vi "MultiDeviceDServer.vi"() -> ()   [LabVIEW 2014, in "examples.lvlib"]
uses:
  examples.lvlib
  vis/tango_vi.llb/_DServerClientRequest.ctl
  vis/tango_vi.llb/_DServerClientRequestType.ctl
  vis/tango_vi.llb/_DServerClientRequestData.ctl
  vis/tango_vi.llb/_GenericDataBuffer.ctl
  vis/tango_vi.llb/_AttributeDataType_t.ctl
  vis/tango_vi.llb/_TangoState_t.ctl
  vis/tango_vi.llb/_DServerSetStateScalarAttributeValue.vi
  vis/tango_vi.llb/_DServerSetStringScalarAttributeValue.vi
  Common/UtilsRandomInstances/_UtilsRandom2DBoolArray.vi
  vis/tango_vi.llb/_DServerSetBooleanImageAttributeValue.vi
  Common/UtilsRandomInstances/_UtilsRandomBoolValue.vi
  vis/tango_vi.llb/_DServerSetBooleanScalarAttributeValue.vi
  Common/UtilsRandomInstances/_UtilsRandomBoolArray.vi
  vis/tango_vi.llb/_DServerSetBooleanSpectrumAttributeValue.vi
  Common/UtilsRandomInstances/_UtilsRandom2DDBLArray.vi
  vis/tango_vi.llb/_DServerSetDoubleImageAttributeValue.vi
  vis/tango_vi.llb/_DServerSetDoubleScalarAttributeValue.vi
  Common/UtilsRandomInstances/_UtilsRandomDBLArray.vi
  vis/tango_vi.llb/_DServerSetDoubleSpectrumAttributeValue.vi
  Common/UtilsRandomInstances/_UtilsRandom2DSGLArray.vi
  vis/tango_vi.llb/_DServerSetFloatImageAttributeValue.vi
  Common/UtilsRandomInstances/_UtilsRandomSGLArray.vi
  vis/tango_vi.llb/_DServerSetFloatSpectrumAttributeValue.vi
  Common/UtilsRandomInstances/_UtilsRandom2DU64Array.vi
  vis/tango_vi.llb/_DServerSetLong64ImageAttributeValue.vi
  Common/UtilsRandomInstances/_UtilsRandomI64Value.vi
  vis/tango_vi.llb/_DServerSetLong64ScalarAttributeValue.vi
  Common/UtilsRandomInstances/_UtilsRandomI64Array.vi
  vis/tango_vi.llb/_DServerSetLong64SpectrumAttributeValue.vi
  Common/UtilsRandomInstances/_UtilsRandom2DI32Array.vi
  vis/tango_vi.llb/_DServerSetLongImageAttributeValue.vi
  Common/UtilsRandomInstances/_UtilsRandomI32Value.vi
  vis/tango_vi.llb/_DServerSetLongScalarAttributeValue.vi
  Common/UtilsRandomInstances/_UtilsRandomU32Array.vi
  vis/tango_vi.llb/_DServerSetLongSpectrumAttributeValue.vi
  Common/UtilsRandomInstances/_UtilsRandom2DI16Array.vi
  vis/tango_vi.llb/_DServerSetShortImageAttributeValue.vi
  Common/UtilsRandomInstances/_UtilsRandomI16Value.vi
  vis/tango_vi.llb/_DServerSetEnumScalarAttributeValue.vi
  Common/UtilsRandomInstances/_UtilsRandomI16Array.vi
  vis/tango_vi.llb/_DServerSetShortSpectrumAttributeValue.vi
  vis/tango_vi.llb/_DServerSetStateImageAttributeValue.vi
  vis/tango_vi.llb/_DServerSetStateSpectrumAttributeValue.vi
  vis/tango_vi.llb/_DServerSetStringImageAttributeValue.vi
  vis/tango_vi.llb/_DServerSetStringSpectrumAttributeValue.vi
  Common/UtilsRandomInstances/_UtilsRandom2DU8Array.vi
  vis/tango_vi.llb/_DServerSetUCharImageAttributeValue.vi
  Common/UtilsRandomInstances/_UtilsRandomU8Value.vi
  vis/tango_vi.llb/_DServerSetUCharScalarAttributeValue.vi
  Common/UtilsRandomInstances/_UtilsRandomU8Array.vi
  vis/tango_vi.llb/_DServerSetUCharSpectrumAttributeValue.vi
  Common/UtilsRandomInstances/_UtilsRandom2DI64Array.vi
  Common/UtilsRandomInstances/_UtilsRandomU64Value.vi
  vis/tango_vi.llb/_DServerSetULong64ScalarAttributeValue.vi
  Common/UtilsRandomInstances/_UtilsRandomU64Array.vi
  vis/tango_vi.llb/_DServerSetULong64SpectrumAttributeValue.vi
  Common/UtilsRandomInstances/_UtilsRandom2DU32Array.vi
  vis/tango_vi.llb/_DServerSetULongImageAttributeValue.vi
  Common/UtilsRandomInstances/_UtilsRandomU32Value.vi
  vis/tango_vi.llb/_DServerSetULongScalarAttributeValue.vi
  Common/UtilsRandomInstances/_UtilsRandomI32Array.vi
  vis/tango_vi.llb/_DServerSetULongSpectrumAttributeValue.vi
  Common/UtilsRandomInstances/_UtilsRandom2DU16Array.vi
  vis/tango_vi.llb/_DServerSetUShortImageAttributeValue.vi
  Common/UtilsRandomInstances/_UtilsRandomU16Value.vi
  vis/tango_vi.llb/_DServerSetUShortScalarAttributeValue.vi
  Common/UtilsRandomInstances/_UtilsRandomU16Array.vi
  vis/tango_vi.llb/_DServerSetUShortSpectrumAttributeValue.vi
  vis/tango_vi.llb/tango.lvlib
panel:
  out "Tango Device State 2.1":T1=enum."UNKNOWN"
  out "Tango Device State 1.2":T1=enum."UNKNOWN"
  in  "devDoubleScalar":dbl(knob)=70.0 scale=0.0..100.0
  out "labview/device/2.1":T2={"Request Id"=0, "Source Id"=0, "Request Type"=enum."UNKNOWN_REQUEST", "Device Class Name"="unspecified/device/name", "Device Name"="unspecified/device/name", "Cmd or Attr Name"="unspecified_cmd_or_attr_name", "Client Request Data"={"write attribute value"={"dimx"=0, "dimy"=0, "data"=[], "data_type"=enum."UNKNOWN_DATA_TYPE"}, "exec. command argin"={"num data"=[], "str data"=[]}}}
  in  "devDoubleScalar":dbl(knob)=50.0 scale=0.0..100.0
  out "Tango Device State 1.1":T1=enum."UNKNOWN"
  out "labview/device/1.2":T2={"Request Id"=0, "Source Id"=0, "Request Type"=enum."UNKNOWN_REQUEST", "Device Class Name"="unspecified/device/name", "Device Name"="unspecified/device/name", "Cmd or Attr Name"="unspecified_cmd_or_attr_name", "Client Request Data"={"write attribute value"={"dimx"=0, "dimy"=0, "data"=[], "data_type"=enum."UNKNOWN_DATA_TYPE"}, "exec. command argin"={"num data"=[], "str data"=[]}}}
  out "labview/device/1.1":T2={"Request Id"=0, "Source Id"=0, "Request Type"=enum."UNKNOWN_REQUEST", "Device Class Name"="unspecified/device/name", "Device Name"="unspecified/device/name", "Cmd or Attr Name"="unspecified_cmd_or_attr_name", "Client Request Data"={"write attribute value"={"dimx"=0, "dimy"=0, "data"=[], "data_type"=enum."UNKNOWN_DATA_TYPE"}, "exec. command argin"={"num data"=[], "str data"=[]}}}
  in  "Tango Client Request":T2={"Request Id"=0, "Source Id"=0, "Request Type"=enum."UNKNOWN_REQUEST", "Device Class Name"="unspecified_class_name", "Device Name"="unspecified/device/name", "Cmd or Attr Name"="unspecified_cmd_or_attr_name", "Client Request Data"={"write attribute value"={"dimx"=0, "dimy"=0, "data"=[], "data_type"=enum."UNKNOWN_DATA_TYPE"}, "exec. command argin"={"num data"=[], "str data"=[]}}}
  out "Device List":string[](array[string])
  in  "Instance Name":string="1"
  in  "Executable Name":string="LabviewMultiDeviceDServer"
  in  "devDoubleScalar":dbl(knob)=30.0 scale=0.0..100.0
  in  "?":bool
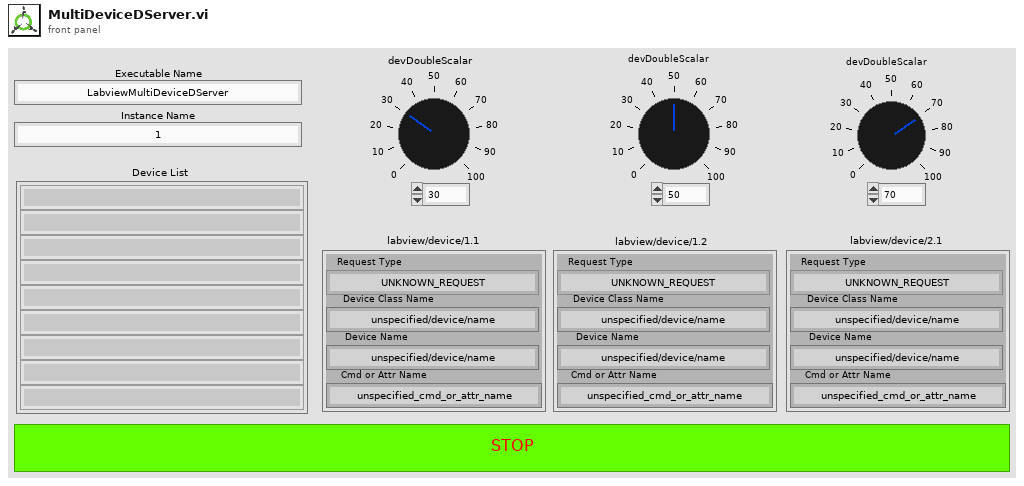
[diagram p1: front panel]
types:
  T1 = typedef "tango.lvlib/_TangoState_t.ctl" = enum32{"ON", "OFF", "CLOSE", "OPEN", "INSERT", "EXTRACT", "MOVING", "STANDBY", "FAULT", "INIT", "RUNNING", "ALARM", "DISABLE", "UNKNOWN"}
  T2 = typedef "tango.lvlib/_DServerClientRequest.ctl" = cluster{"Request Id":u32, "Source Id":u32, "Request Type":T3, "Device Class Name":string, "Device Name":string, "Cmd or Attr Name":string, "Client Request Data":T4}
  T3 = typedef "tango.lvlib/_DServerClientRequestType.ctl" = enum16{"EXEC_CMD", "READ_ATTR", "WRITE_ATTR", "UNKNOWN_REQUEST"}
  T4 = typedef "tango.lvlib/_DServerClientRequestData.ctl" = cluster{"write attribute value":T5, "exec. command argin":cluster{"num data":u8[], "str data":string[]}}
  T5 = typedef "tango.lvlib/_GenericDataBuffer.ctl" = cluster{"dimx":u32, "dimy":u32, "data":u8[], "data_type":T6}
  T6 = typedef "tango.lvlib/_AttributeDataType_t.ctl" = enum16{"STATE_SCA", "STATE_SPE", "STATE_IMG", "STRING_SCA", "STRING_SPE", "STRING_IMG", "BOOL_SCA", "BOOL_SPE", "BOOL_IMG", "UCHAR_SCA", "UCHAR_SPE", "UCHAR_IMG", "SHORT_SCA", "SHORT_SPE", "SHORT_IMG", "USHORT_SCA", "USHORT_SPE", "USHORT_IMG", "LONG_SCA", "LONG_SPE", "LONG_IMG", "ULONG_SCA", "ULONG_SPE", "ULONG_IMG", "LONG64_SCA", "LONG64_SPE", "LONG64_IMG", "ULONG64_SCA", "ULONG64_SPE", "ULONG64_IMG", "FLOAT_SCA", "FLOAT_SPE", "FLOAT_IMG", "DOUBLE_SCA", "DOUBLE_SPE", "DOUBLE_IMG", "ENUM_SCA", "UNKNOWN_DATA_TYPE"}
  T7 = typedef "tango.lvlib/_DServerEvent.ctl" = cluster{"event registration refnum":refnum<event-registration>, "user event out":refnum<user-event>}
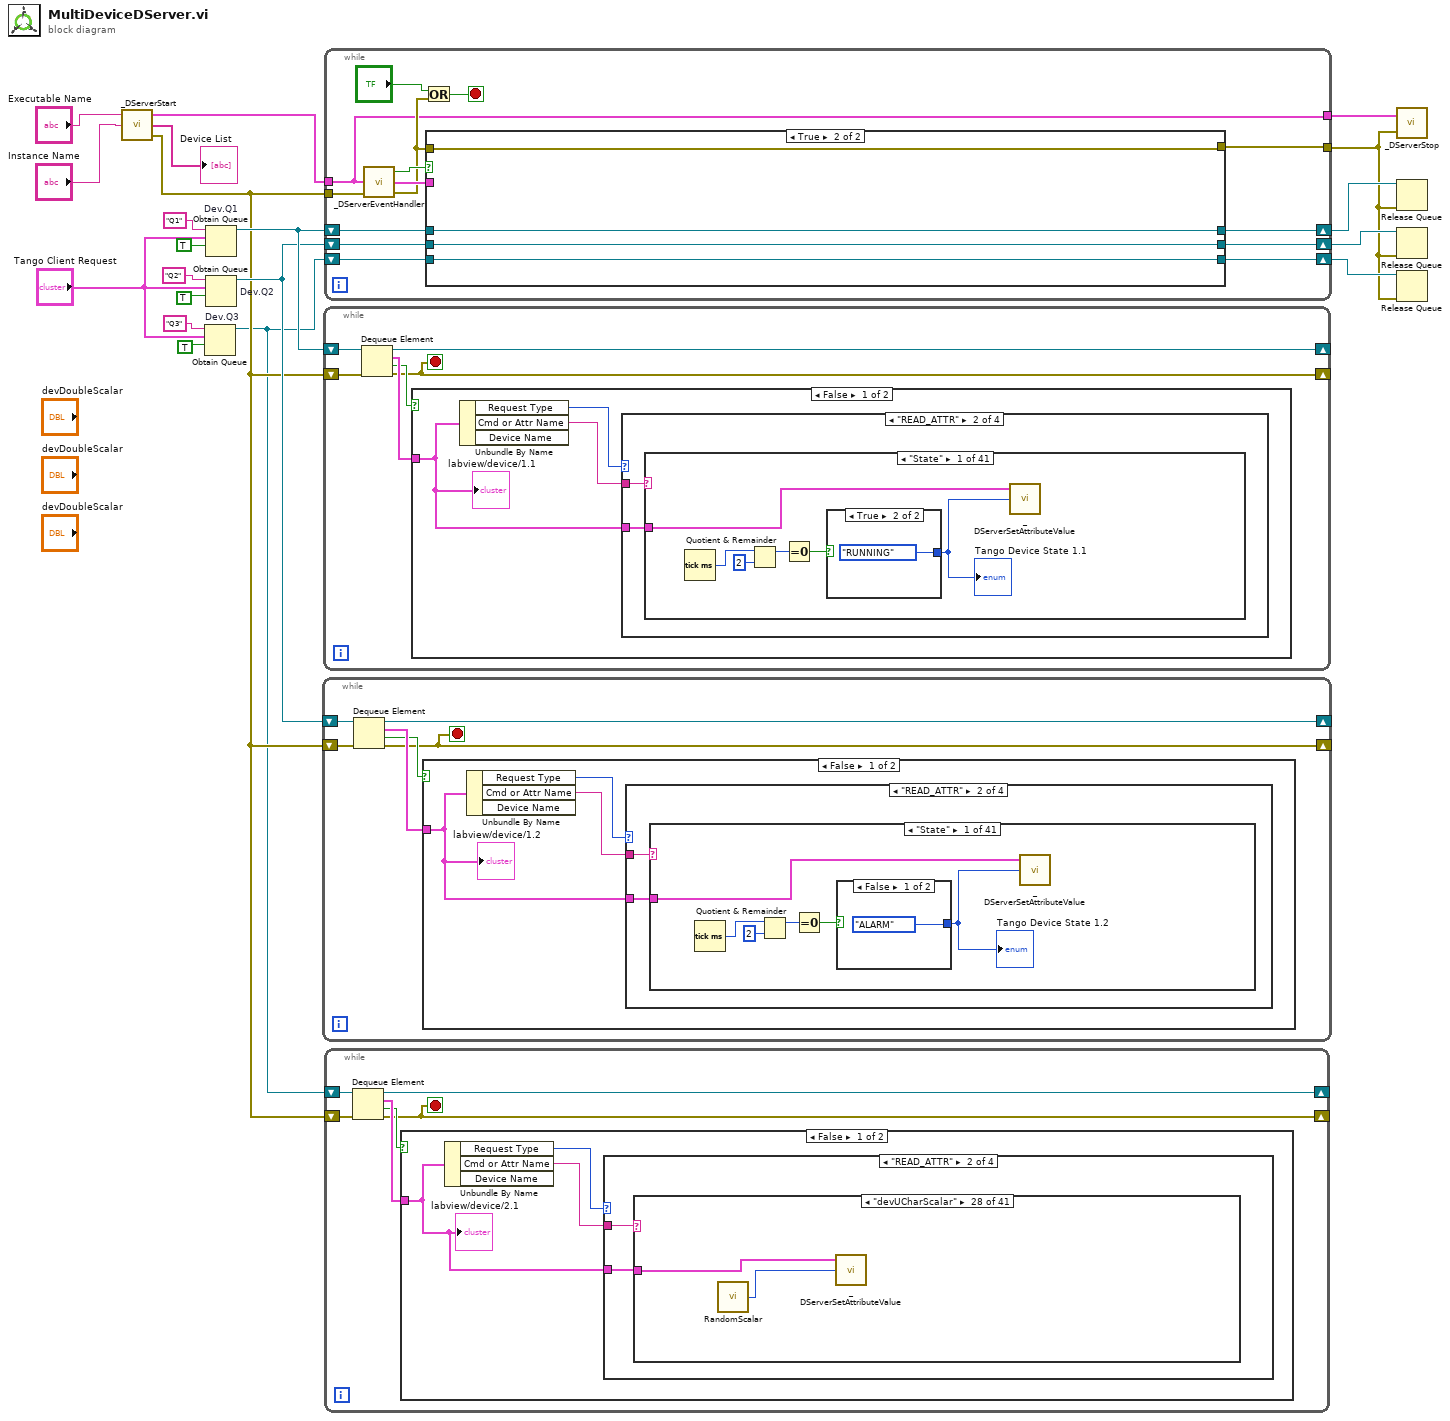
[diagram p0: block diagram]
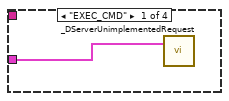
[diagram p2: hidden frame]
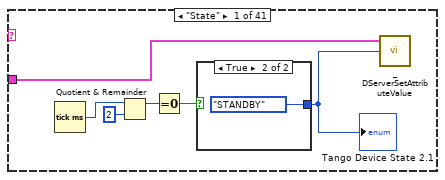
[diagram p3: hidden frame]
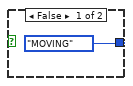
[diagram p4: hidden frame]
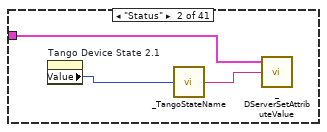
[diagram p5: hidden frame]
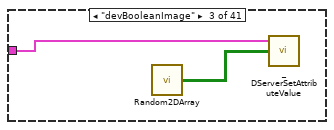
[diagram p6: hidden frame]
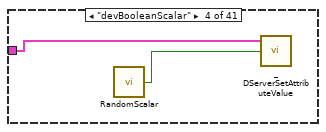
[diagram p7: hidden frame]
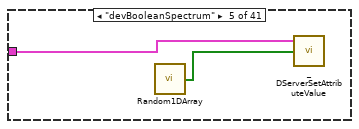
[diagram p8: hidden frame]
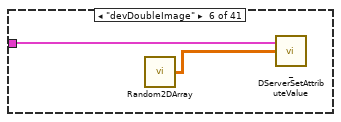
[diagram p9: hidden frame]
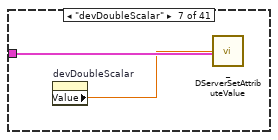
[diagram p10: hidden frame]
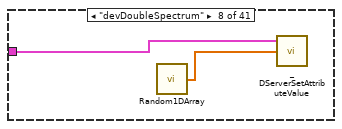
[diagram p11: hidden frame]
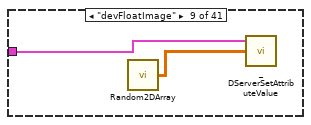
[diagram p12: hidden frame]
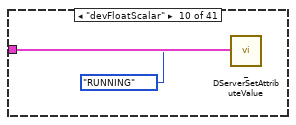
[diagram p13: hidden frame]
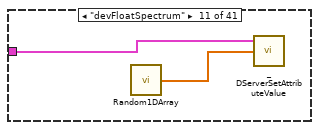
[diagram p14: hidden frame]
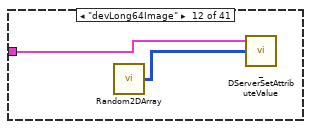
[diagram p15: hidden frame]
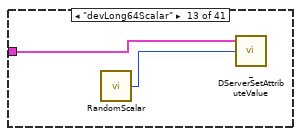
[diagram p16: hidden frame]
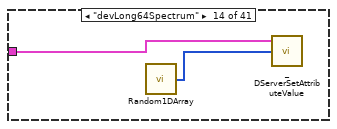
[diagram p17: hidden frame]
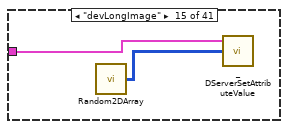
[diagram p18: hidden frame]
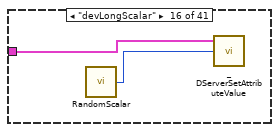
[diagram p19: hidden frame]
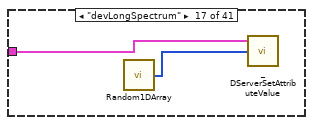
[diagram p20: hidden frame]
diagram:
  n1 = call "_DServerStart.vi"("instance name"="Instance Name", "executable name"="Executable Name") -> ("error out"=w2:errorcluster, "device_list"=→"Device List":string[], "dserver evt."=w5:T7)  [unwired: 1 in]
  n2 = Obtain Queue "Dev.Q3"(name (unnamed)="Q3", element data type="Tango Client Request", create if not found? (T)=TRUE) -> (queue out=w1:refnum<queue>)  [unwired: 2 in, 2 out]
  n3 = Obtain Queue "Dev.Q1"(name (unnamed)="Q1", element data type="Tango Client Request", create if not found? (T)=TRUE) -> (queue out=w18:refnum<queue>)  [unwired: 2 in, 2 out]
  n4 = Obtain Queue "Dev.Q2"(name (unnamed)="Q2", element data type="Tango Client Request", create if not found? (T)=TRUE) -> (queue out=w14:refnum<queue>)  [unwired: 2 in, 2 out]
  n5 = while {
    shift-right: [w21] -> _
    shift-left: w2 -> [w22]
    shift-right: [w23] -> _
    shift-left: w14 -> [w26]
    stop <- w21 stop-if-true
    n6 = Dequeue Element(queue=w26, error in (no error)=w22) -> (queue out=w23:refnum<queue>, element=w25:T2, timed out?=w24:bool, error out=w21:errorcluster)  [unwired: 1 in]
    n7 = case shown="False" w24 {
      tunnel: w25 -> [w27 _]
      frame False {
        n8 = Unbundle By Name(w27) -> ("Request Type"=w28:T3, "Cmd or Attr Name"=w29:string)  [unwired: 1 out]
        n9 = case shown="\"READ_ATTR\"" w28 {
          tunnel: w29 -> [_ w32 _ _]
          tunnel: w27 -> [w30 w31 w140 w141]
          frame "EXEC_CMD" {
            n10 = call "_DServerUnimplementedRequest.vi"("client request"=w30) -> ()  [unwired: 2 in, 1 out]
          }
          frame "READ_ATTR" {
            n11 = case shown="\"State\"" w32 {
              tunnel: w31 -> [w34 w42 w45 w47 w49 w51 w53 w55 w57 w58 w61 w63 w65 w67 w69 w71 w73 w75 w77 w79 w82 w85 w95 w102 w105 w110 w112 w114 w116 w118 w120 w122 w124 w126 w128 w130 w132 w134 w135 _ w139]
              frame "State" {
                n12 = Tick Count (ms)() -> (millisecond timer value=w35:u32)
                n13 = Quotient & Remainder(x=w35, y=u32 2) -> (x-y*floor(x/y)=w37:u32)  [unwired: 1 out]
                n14 = Equal To 0?(x=w37) -> (x = 0?=w36:bool)
                n15 = case shown="False" w36 {
                  tunnel: [_TangoState_t."ALARM" ("Tango Device State") _TangoState_t."FAULT" ("Tango Device State")] -> w33
                  frame False {
                  }
                  frame True {
                  }
                }
                "Tango Device State 1.2" <- w33
                n16 = call-poly "_DServerSetAttributeValue.vi"("value"=w33, "client request"=w34) -> ()  [unwired: 3 in, 1 out]
              }
              frame "Status" {
                n17 = property on="Tango Device State 1.2" class="Enum (strict)"() -> ("Value"=w41:T1)  [unwired: 2 in, 2 out]
                n18 = call "_TangoStateName.vi"("State"=w41) -> ("State Name"=w43:string)
                n19 = call-poly "_DServerSetAttributeValue.vi"("value"=w43, "client request"=w42) -> ()  [unwired: 3 in, 1 out]
              }
              frame "devBooleanImage" {
                n20 = call-poly "Random2DArray.vi"() -> ("random array"=w44:bool[][])  [unwired: 2 in]
                n21 = call-poly "_DServerSetAttributeValue.vi"("value"=w44, "client request"=w45) -> ()  [unwired: 3 in, 1 out]
              }
              frame "devBooleanScalar" {
                n22 = call-poly "RandomScalar.vi"() -> ("random value"=w46:bool)  [unwired: 1 in]
                n23 = call-poly "_DServerSetAttributeValue.vi"(4:w46, "client request"=w47) -> ()  [unwired: 3 in, 1 out]
              }
              frame "devBooleanSpectrum" {
                n24 = call-poly "Random1DArray.vi"() -> ("array"=w48:bool[])  [unwired: 2 in]
                n25 = call-poly "_DServerSetAttributeValue.vi"("value"=w48, "client request"=w49) -> ()  [unwired: 3 in, 1 out]
              }
              frame "devDoubleImage" {
                n26 = call-poly "Random2DArray.vi"() -> ("random array"=w50:dbl[][])  [unwired: 2 in]
                n27 = call-poly "_DServerSetAttributeValue.vi"("value"=w50, "client request"=w51) -> ()  [unwired: 3 in, 1 out]
              }
              frame "devDoubleScalar" {
                n28 = property on="devDoubleScalar" class="Knob (strict)"() -> ("Value"=w52:dbl)  [unwired: 2 in, 2 out]
                n29 = call-poly "_DServerSetAttributeValue.vi"("value"=w52, "client request"=w53) -> ()  [unwired: 3 in, 1 out]
              }
              frame "devDoubleSpectrum" {
                n30 = call-poly "Random1DArray.vi"() -> ("array"=w54:dbl[])  [unwired: 2 in]
                n31 = call-poly "_DServerSetAttributeValue.vi"("value"=w54, "client request"=w55) -> ()  [unwired: 3 in, 1 out]
              }
              frame "devFloatImage" {
                n32 = call-poly "Random2DArray.vi"() -> ("random array"=w56:sgl[][])  [unwired: 2 in]
                n33 = call-poly "_DServerSetAttributeValue.vi"("value"=w56, "client request"=w57) -> ()  [unwired: 3 in, 1 out]
              }
              frame "devFloatScalar" {
                n34 = call-poly "_DServerSetAttributeValue.vi"("value"=_TangoState_t."RUNNING" ("Tango Device State"), "client request"=w58) -> ()  [unwired: 3 in, 1 out]
              }
              frame "devFloatSpectrum" {
                n35 = call-poly "Random1DArray.vi"() -> ("array"=w60:sgl[])  [unwired: 2 in]
                n36 = call-poly "_DServerSetAttributeValue.vi"("value"=w60, "client request"=w61) -> ()  [unwired: 3 in, 1 out]
              }
              frame "devLong64Image" {
                n37 = call-poly "Random2DArray.vi"() -> ("random array"=w62:i64[][])  [unwired: 2 in]
                n38 = call-poly "_DServerSetAttributeValue.vi"("value"=w62, "client request"=w63) -> ()  [unwired: 3 in, 1 out]
              }
              frame "devLong64Scalar" {
                n39 = call-poly "RandomScalar.vi"() -> ("random value"=w64:i64)  [unwired: 1 in]
                n40 = call-poly "_DServerSetAttributeValue.vi"("value"=w64, "client request"=w65) -> ()  [unwired: 3 in, 1 out]
              }
              frame "devLong64Spectrum" {
                n41 = call-poly "Random1DArray.vi"() -> ("array"=w66:i64[])  [unwired: 2 in]
                n42 = call-poly "_DServerSetAttributeValue.vi"("value"=w66, "client request"=w67) -> ()  [unwired: 3 in, 1 out]
              }
              frame "devLongImage" {
                n43 = call-poly "Random2DArray.vi"() -> ("random array"=w68:i32[][])  [unwired: 2 in]
                n44 = call-poly "_DServerSetAttributeValue.vi"("value"=w68, "client request"=w69) -> ()  [unwired: 3 in, 1 out]
              }
              frame "devLongScalar" {
                n45 = call-poly "RandomScalar.vi"() -> ("random value"=w70:i32)  [unwired: 1 in]
                n46 = call-poly "_DServerSetAttributeValue.vi"("value"=w70, "client request"=w71) -> ()  [unwired: 3 in, 1 out]
              }
              frame "devLongSpectrum" {
                n47 = call-poly "Random1DArray.vi"() -> ("array"=w72:i32[])  [unwired: 2 in]
                n48 = call-poly "_DServerSetAttributeValue.vi"("value"=w72, "client request"=w73) -> ()  [unwired: 3 in, 1 out]
              }
              frame "devShortImage" {
                n49 = call-poly "Random2DArray.vi"() -> ("random array"=w74:i16[][])  [unwired: 2 in]
                n50 = call-poly "_DServerSetAttributeValue.vi"("value"=w74, "client request"=w75) -> ()  [unwired: 3 in, 1 out]
              }
              frame "devShortScalar" {
                n51 = call-poly "RandomScalar.vi"() -> ("random value"=w76:i16)  [unwired: 1 in]
                n52 = call-poly "_DServerSetAttributeValue.vi"("value"=w76, "client request"=w77) -> ()  [unwired: 3 in, 1 out]
              }
              frame "devShortSpectrum" {
                n53 = call-poly "Random1DArray.vi"() -> ("array"=w78:i16[])  [unwired: 2 in]
                n54 = call-poly "_DServerSetAttributeValue.vi"("value"=w78, "client request"=w79) -> ()  [unwired: 3 in, 1 out]
              }
              frame "devStateImage" {
                n55 = property on="Tango Device State 1.2" class="Enum (strict)"() -> ("Value"=w81:T1)  [unwired: 2 in, 2 out]
                n56 = Initialize Array(w81, 32 ("dimension size"), 32 ("dimension size")) -> (w80:T1[][])
                n57 = call-poly "_DServerSetAttributeValue.vi"("value"=w80, "client request"=w82) -> ()  [unwired: 3 in, 1 out]
              }
              frame "devStateScalar" {
                n58 = Tick Count (ms)() -> (millisecond timer value=w87:u32)
                n59 = Quotient & Remainder(x=w87, y=u32 2) -> (x-y*floor(x/y)=w89:u32)  [unwired: 1 out]
                n60 = Equal To 0?(x=w89) -> (x = 0?=w88:bool)
                n61 = case shown="False" w88 {
                  tunnel: [_TangoState_t."STANDBY" ("Tango Device State") _TangoState_t."RUNNING" ("Tango Device State")] -> w86
                  frame False {
                  }
                  frame True {
                  }
                }
                n62 = call-poly "_DServerSetAttributeValue.vi"("value"=w86, "client request"=w85) -> ()  [unwired: 3 in, 1 out]
              }
              frame "devStateSpectrum" {
                n63 = property on="Tango Device State 1.2" class="Enum (strict)"() -> ("Value"=w94:T1)  [unwired: 2 in, 2 out]
                n64 = Initialize Array(w94, 32 ("dimension size")) -> (w93:T1[])
                n65 = call-poly "_DServerSetAttributeValue.vi"("value"=w93, "client request"=w95) -> ()  [unwired: 3 in, 1 out]
              }
              frame "devStringImage" {
                n66 = call "RandomValue.vi"() -> ("random value"=w100:dbl)  [unwired: 1 in]
                n67 = Number To Hexadecimal String(2:w100) -> (0:w99:string)  [unwired: 1 in]
                n68 = Initialize Array(w99, 32 ("dimension size"), 32 ("dimension size")) -> (w98:string[][])
                n69 = call-poly "_DServerSetAttributeValue.vi"("value"=w98, "client request"=w102) -> ()  [unwired: 3 in, 1 out]
              }
              frame "devStringScalar" {
                n70 = call "RandomValue.vi"() -> ("random value"=w104:dbl)  [unwired: 1 in]
                n71 = Number To Hexadecimal String(2:w104) -> (0:w103:string)  [unwired: 1 in]
                n72 = call-poly "_DServerSetAttributeValue.vi"("value"=w103, "client request"=w105) -> ()  [unwired: 3 in, 1 out]
              }
              frame "devStringSpectrum" {
                n73 = call "RandomValue.vi"() -> ("random value"=w108:dbl)  [unwired: 1 in]
                n74 = Number To Hexadecimal String(2:w108) -> (0:w107:string)  [unwired: 1 in]
                n75 = Initialize Array(w107, 32 ("dimension size")) -> (w106:string[])
                n76 = call-poly "_DServerSetAttributeValue.vi"("value"=w106, "client request"=w110) -> ()  [unwired: 3 in, 1 out]
              }
              frame "devUCharImage" {
                n77 = call-poly "Random2DArray.vi"() -> ("random array"=w111:u8[][])  [unwired: 2 in]
                n78 = call-poly "_DServerSetAttributeValue.vi"("value"=w111, "client request"=w112) -> ()  [unwired: 3 in, 1 out]
              }
              frame "devUCharScalar" {
                n79 = call-poly "RandomScalar.vi"() -> ("random value"=w113:u8)  [unwired: 1 in]
                n80 = call-poly "_DServerSetAttributeValue.vi"("value"=w113, "client request"=w114) -> ()  [unwired: 3 in, 1 out]
              }
              frame "devUCharSpectrum" {
                n81 = call-poly "Random1DArray.vi"() -> ("array"=w115:u8[])  [unwired: 2 in]
                n82 = call-poly "_DServerSetAttributeValue.vi"("value"=w115, "client request"=w116) -> ()  [unwired: 3 in, 1 out]
              }
              frame "devULong64Image" {
                n83 = call-poly "Random2DArray.vi"() -> ("random array"=w117:i64[][])  [unwired: 2 in]
                n84 = call-poly "_DServerSetAttributeValue.vi"("value"=w117, "client request"=w118) -> ()  [unwired: 3 in, 1 out]
              }
              frame "devULong64Scalar" {
                n85 = call-poly "RandomScalar.vi"() -> ("random value"=w119:u64)  [unwired: 1 in]
                n86 = call-poly "_DServerSetAttributeValue.vi"("value"=w119, "client request"=w120) -> ()  [unwired: 3 in, 1 out]
              }
              frame "devULong64Spectrum" {
                n87 = call-poly "Random1DArray.vi"() -> ("array"=w121:u64[])  [unwired: 2 in]
                n88 = call-poly "_DServerSetAttributeValue.vi"("value"=w121, "client request"=w122) -> ()  [unwired: 3 in, 1 out]
              }
              frame "devULongImage" {
                n89 = call-poly "Random2DArray.vi"() -> ("random array"=w123:u32[][])  [unwired: 2 in]
                n90 = call-poly "_DServerSetAttributeValue.vi"("value"=w123, "client request"=w124) -> ()  [unwired: 3 in, 1 out]
              }
              frame "devULongScalar" {
                n91 = call-poly "RandomScalar.vi"() -> ("random value"=w125:u32)  [unwired: 1 in]
                n92 = call-poly "_DServerSetAttributeValue.vi"("value"=w125, "client request"=w126) -> ()  [unwired: 3 in, 1 out]
              }
              frame "devULongSpectrum" {
                n93 = call-poly "Random1DArray.vi"() -> ("array"=w127:u32[])  [unwired: 2 in]
                n94 = call-poly "_DServerSetAttributeValue.vi"("value"=w127, "client request"=w128) -> ()  [unwired: 3 in, 1 out]
              }
              frame "devUShortImage" {
                n95 = call-poly "Random2DArray.vi"() -> ("random array"=w129:u16[][])  [unwired: 2 in]
                n96 = call-poly "_DServerSetAttributeValue.vi"("value"=w129, "client request"=w130) -> ()  [unwired: 3 in, 1 out]
              }
              frame "devUShortScalar" {
                n97 = call-poly "RandomScalar.vi"() -> ("random value"=w131:u16)  [unwired: 1 in]
                n98 = call-poly "_DServerSetAttributeValue.vi"("value"=w131, "client request"=w132) -> ()  [unwired: 3 in, 1 out]
              }
              frame "devUShortSpectrum" {
                n99 = call-poly "Random1DArray.vi"() -> ("array"=w133:u16[])  [unwired: 2 in]
                n100 = call-poly "_DServerSetAttributeValue.vi"("value"=w133, "client request"=w134) -> ()  [unwired: 3 in, 1 out]
              }
              frame "slowReplyAttribute" {
                n101 = stacked-sequence {
                  tunnel: w135 -> [_ w138]
                  frame #0 {
                    # "simulate a slow reply \ngenerating a client \nrequest timeout"
                    n102 = Wait (ms)(milliseconds to wait=u32 3500) -> ()  [unwired: 1 out]
                  }
                  frame #1 {
                    # "simulate a slow reply \ngenerating a client \nrequest timeout"
                    n103 = call-poly "Random1DArray.vi"() -> ("array"=w137:u8[])  [unwired: 2 in]
                    n104 = call-poly "_DServerSetAttributeValue.vi"("value"=w137, "client request"=w138) -> ()  [unwired: 3 in, 1 out]
                  }
                }
              }
              frame "noReplyAttribute" {
                # "we voluntarily don't reply to this request in order to\nobserve the behavior of the tango binding to such a \nsituation - we expect the waiter (i.e. the thread handling \nthe client request to timeout and leave the place) - the \ntango device will block (i.e. will not be able to handle \nanother request) until the timeout expires - we consequently understand easily why we should reply to any single request - the _DServerUnimplementedRequest.vi can be temporary used to deal with \"not yet implemented\" features - see the \"unhandledAttribute\" case for an example"
              }
              frame "unHandledAttribute", Default {
                n105 = call "_DServerUnimplementedRequest.vi"("client request"=w139) -> ()  [unwired: 2 in, 1 out]
              }
            }
          }
          frame "WRITE_ATTR" {
            n106 = call "_DServerUnimplementedRequest.vi"("client request"=w140) -> ()  [unwired: 2 in, 1 out]
          }
          frame "UNKNOWN_REQUEST", Default {
            n107 = call "_DServerUnimplementedRequest.vi"("client request"=w141) -> ()  [unwired: 2 in, 1 out]
          }
        }
        "labview/device/1.2" <- w27
      }
      frame True {
      }
    }
  }
  n108 = while {
    shift-right: [w142] -> _
    shift-left: w2 -> [w143]
    shift-right: [w144] -> _
    shift-left: w18 -> [w147]
    stop <- w142 stop-if-true
    n109 = Dequeue Element(queue=w147, error in (no error)=w143) -> (queue out=w144:refnum<queue>, element=w146:T2, timed out?=w145:bool, error out=w142:errorcluster)  [unwired: 1 in]
    n110 = case shown="False" w145 {
      tunnel: w146 -> [w148 _]
      frame False {
        n111 = Unbundle By Name(w148) -> ("Request Type"=w149:T3, "Cmd or Attr Name"=w150:string)  [unwired: 1 out]
        n112 = case shown="\"READ_ATTR\"" w149 {
          tunnel: w150 -> [_ w153 _ _]
          tunnel: w148 -> [w151 w152 w261 w262]
          frame "EXEC_CMD" {
            n113 = call "_DServerUnimplementedRequest.vi"("client request"=w151) -> ()  [unwired: 2 in, 1 out]
          }
          frame "READ_ATTR" {
            n114 = case shown="\"State\"" w153 {
              tunnel: w152 -> [w155 w163 w166 w168 w170 w172 w174 w176 w178 w180 w182 w184 w186 w188 w190 w192 w194 w196 w198 w200 w203 w206 w217 w223 w226 w231 w233 w235 w237 w239 w241 w243 w245 w247 w249 w251 w253 w255 w256 _ w260]
              frame "State" {
                n115 = Tick Count (ms)() -> (millisecond timer value=w156:u32)
                n116 = Quotient & Remainder(x=w156, y=u32 2) -> (x-y*floor(x/y)=w158:u32)  [unwired: 1 out]
                n117 = Equal To 0?(x=w158) -> (x = 0?=w157:bool)
                n118 = case shown="True" w157 {
                  tunnel: [_TangoState_t."STANDBY" ("Tango Device State") _TangoState_t."RUNNING" ("Tango Device State")] -> w154
                  frame False {
                  }
                  frame True {
                  }
                }
                "Tango Device State 1.1" <- w154
                n119 = call-poly "_DServerSetAttributeValue.vi"("value"=w154, "client request"=w155) -> ()  [unwired: 3 in, 1 out]
              }
              frame "Status" {
                n120 = property on="Tango Device State 1.1" class="Enum (strict)"() -> ("Value"=w162:T1)  [unwired: 2 in, 2 out]
                n121 = call "_TangoStateName.vi"("State"=w162) -> ("State Name"=w164:string)
                n122 = call-poly "_DServerSetAttributeValue.vi"("value"=w164, "client request"=w163) -> ()  [unwired: 3 in, 1 out]
              }
              frame "devBooleanImage" {
                n123 = call-poly "Random2DArray.vi"() -> ("random array"=w165:bool[][])  [unwired: 2 in]
                n124 = call-poly "_DServerSetAttributeValue.vi"("value"=w165, "client request"=w166) -> ()  [unwired: 3 in, 1 out]
              }
              frame "devBooleanScalar" {
                n125 = call-poly "RandomScalar.vi"() -> ("random value"=w167:bool)  [unwired: 1 in]
                n126 = call-poly "_DServerSetAttributeValue.vi"(4:w167, "client request"=w168) -> ()  [unwired: 3 in, 1 out]
              }
              frame "devBooleanSpectrum" {
                n127 = call-poly "Random1DArray.vi"() -> ("array"=w169:bool[])  [unwired: 2 in]
                n128 = call-poly "_DServerSetAttributeValue.vi"("value"=w169, "client request"=w170) -> ()  [unwired: 3 in, 1 out]
              }
              frame "devDoubleImage" {
                n129 = call-poly "Random2DArray.vi"() -> ("random array"=w171:dbl[][])  [unwired: 2 in]
                n130 = call-poly "_DServerSetAttributeValue.vi"("value"=w171, "client request"=w172) -> ()  [unwired: 3 in, 1 out]
              }
              frame "devDoubleScalar" {
                n131 = property on="devDoubleScalar" class="Knob (strict)"() -> ("Value"=w173:dbl)  [unwired: 2 in, 2 out]
                n132 = call-poly "_DServerSetAttributeValue.vi"("value"=w173, "client request"=w174) -> ()  [unwired: 3 in, 1 out]
              }
              frame "devDoubleSpectrum" {
                n133 = call-poly "Random1DArray.vi"() -> ("array"=w175:dbl[])  [unwired: 2 in]
                n134 = call-poly "_DServerSetAttributeValue.vi"("value"=w175, "client request"=w176) -> ()  [unwired: 3 in, 1 out]
              }
              frame "devFloatImage" {
                n135 = call-poly "Random2DArray.vi"() -> ("random array"=w177:sgl[][])  [unwired: 2 in]
                n136 = call-poly "_DServerSetAttributeValue.vi"("value"=w177, "client request"=w178) -> ()  [unwired: 3 in, 1 out]
              }
              frame "devFloatScalar" {
                n137 = call-poly "_DServerSetAttributeValue.vi"("value"=_TangoState_t."RUNNING" ("Tango Device State"), "client request"=w180) -> ()  [unwired: 3 in, 1 out]
              }
              frame "devFloatSpectrum" {
                n138 = call-poly "Random1DArray.vi"() -> ("array"=w181:sgl[])  [unwired: 2 in]
                n139 = call-poly "_DServerSetAttributeValue.vi"("value"=w181, "client request"=w182) -> ()  [unwired: 3 in, 1 out]
              }
              frame "devLong64Image" {
                n140 = call-poly "Random2DArray.vi"() -> ("random array"=w183:i64[][])  [unwired: 2 in]
                n141 = call-poly "_DServerSetAttributeValue.vi"("value"=w183, "client request"=w184) -> ()  [unwired: 3 in, 1 out]
              }
              frame "devLong64Scalar" {
                n142 = call-poly "RandomScalar.vi"() -> ("random value"=w185:i64)  [unwired: 1 in]
                n143 = call-poly "_DServerSetAttributeValue.vi"("value"=w185, "client request"=w186) -> ()  [unwired: 3 in, 1 out]
              }
              frame "devLong64Spectrum" {
                n144 = call-poly "Random1DArray.vi"() -> ("array"=w187:i64[])  [unwired: 2 in]
                n145 = call-poly "_DServerSetAttributeValue.vi"("value"=w187, "client request"=w188) -> ()  [unwired: 3 in, 1 out]
              }
              frame "devLongImage" {
                n146 = call-poly "Random2DArray.vi"() -> ("random array"=w189:i32[][])  [unwired: 2 in]
                n147 = call-poly "_DServerSetAttributeValue.vi"("value"=w189, "client request"=w190) -> ()  [unwired: 3 in, 1 out]
              }
              frame "devLongScalar" {
                n148 = call-poly "RandomScalar.vi"() -> ("random value"=w191:i32)  [unwired: 1 in]
                n149 = call-poly "_DServerSetAttributeValue.vi"("value"=w191, "client request"=w192) -> ()  [unwired: 3 in, 1 out]
              }
              frame "devLongSpectrum" {
                n150 = call-poly "Random1DArray.vi"() -> ("array"=w193:i32[])  [unwired: 2 in]
                n151 = call-poly "_DServerSetAttributeValue.vi"("value"=w193, "client request"=w194) -> ()  [unwired: 3 in, 1 out]
              }
              frame "devShortImage" {
                n152 = call-poly "Random2DArray.vi"() -> ("random array"=w195:i16[][])  [unwired: 2 in]
                n153 = call-poly "_DServerSetAttributeValue.vi"("value"=w195, "client request"=w196) -> ()  [unwired: 3 in, 1 out]
              }
              frame "devShortScalar" {
                n154 = call-poly "RandomScalar.vi"() -> ("random value"=w197:i16)  [unwired: 1 in]
                n155 = call-poly "_DServerSetAttributeValue.vi"("value"=w197, "client request"=w198) -> ()  [unwired: 3 in, 1 out]
              }
              frame "devShortSpectrum" {
                n156 = call-poly "Random1DArray.vi"() -> ("array"=w199:i16[])  [unwired: 2 in]
                n157 = call-poly "_DServerSetAttributeValue.vi"("value"=w199, "client request"=w200) -> ()  [unwired: 3 in, 1 out]
              }
              frame "devStateImage" {
                n158 = property on="Tango Device State 1.1" class="Enum (strict)"() -> ("Value"=w201:T1)  [unwired: 2 in, 2 out]
                n159 = Initialize Array(w201, 32 ("dimension size"), 32 ("dimension size")) -> (w202:T1[][])
                n160 = call-poly "_DServerSetAttributeValue.vi"("value"=w202, "client request"=w203) -> ()  [unwired: 3 in, 1 out]
              }
              frame "devStateScalar" {
                n161 = Tick Count (ms)() -> (millisecond timer value=w208:u32)
                n162 = Quotient & Remainder(x=w208, y=u32 2) -> (x-y*floor(x/y)=w210:u32)  [unwired: 1 out]
                n163 = Equal To 0?(x=w210) -> (x = 0?=w209:bool)
                n164 = case shown="False" w209 {
                  tunnel: [_TangoState_t."STANDBY" ("Tango Device State") _TangoState_t."RUNNING" ("Tango Device State")] -> w207
                  frame False {
                  }
                  frame True {
                  }
                }
                n165 = call-poly "_DServerSetAttributeValue.vi"("value"=w207, "client request"=w206) -> ()  [unwired: 3 in, 1 out]
              }
              frame "devStateSpectrum" {
                n166 = property on="Tango Device State 1.1" class="Enum (strict)"() -> ("Value"=w216:T1)  [unwired: 2 in, 2 out]
                n167 = Initialize Array(w216, 32 ("dimension size")) -> (w214:T1[])
                n168 = call-poly "_DServerSetAttributeValue.vi"("value"=w214, "client request"=w217) -> ()  [unwired: 3 in, 1 out]
              }
              frame "devStringImage" {
                n169 = call "RandomValue.vi"() -> ("random value"=w221:dbl)  [unwired: 1 in]
                n170 = Number To Hexadecimal String(2:w221) -> (0:w220:string)  [unwired: 1 in]
                n171 = Initialize Array(w220, 32 ("dimension size"), 32 ("dimension size")) -> (w219:string[][])
                n172 = call-poly "_DServerSetAttributeValue.vi"("value"=w219, "client request"=w223) -> ()  [unwired: 3 in, 1 out]
              }
              frame "devStringScalar" {
                n173 = call "RandomValue.vi"() -> ("random value"=w225:dbl)  [unwired: 1 in]
                n174 = Number To Hexadecimal String(2:w225) -> (0:w224:string)  [unwired: 1 in]
                n175 = call-poly "_DServerSetAttributeValue.vi"("value"=w224, "client request"=w226) -> ()  [unwired: 3 in, 1 out]
              }
              frame "devStringSpectrum" {
                n176 = call "RandomValue.vi"() -> ("random value"=w229:dbl)  [unwired: 1 in]
                n177 = Number To Hexadecimal String(2:w229) -> (0:w228:string)  [unwired: 1 in]
                n178 = Initialize Array(w228, 32 ("dimension size")) -> (w227:string[])
                n179 = call-poly "_DServerSetAttributeValue.vi"("value"=w227, "client request"=w231) -> ()  [unwired: 3 in, 1 out]
              }
              frame "devUCharImage" {
                n180 = call-poly "Random2DArray.vi"() -> ("random array"=w232:u8[][])  [unwired: 2 in]
                n181 = call-poly "_DServerSetAttributeValue.vi"("value"=w232, "client request"=w233) -> ()  [unwired: 3 in, 1 out]
              }
              frame "devUCharScalar" {
                n182 = call-poly "RandomScalar.vi"() -> ("random value"=w234:u8)  [unwired: 1 in]
                n183 = call-poly "_DServerSetAttributeValue.vi"("value"=w234, "client request"=w235) -> ()  [unwired: 3 in, 1 out]
              }
              frame "devUCharSpectrum" {
                n184 = call-poly "Random1DArray.vi"() -> ("array"=w236:u8[])  [unwired: 2 in]
                n185 = call-poly "_DServerSetAttributeValue.vi"("value"=w236, "client request"=w237) -> ()  [unwired: 3 in, 1 out]
              }
              frame "devULong64Image" {
                n186 = call-poly "Random2DArray.vi"() -> ("random array"=w238:i64[][])  [unwired: 2 in]
                n187 = call-poly "_DServerSetAttributeValue.vi"("value"=w238, "client request"=w239) -> ()  [unwired: 3 in, 1 out]
              }
              frame "devULong64Scalar" {
                n188 = call-poly "RandomScalar.vi"() -> ("random value"=w240:u64)  [unwired: 1 in]
                n189 = call-poly "_DServerSetAttributeValue.vi"("value"=w240, "client request"=w241) -> ()  [unwired: 3 in, 1 out]
              }
              frame "devULong64Spectrum" {
                n190 = call-poly "Random1DArray.vi"() -> ("array"=w242:u64[])  [unwired: 2 in]
                n191 = call-poly "_DServerSetAttributeValue.vi"("value"=w242, "client request"=w243) -> ()  [unwired: 3 in, 1 out]
              }
              frame "devULongImage" {
                n192 = call-poly "Random2DArray.vi"() -> ("random array"=w244:u32[][])  [unwired: 2 in]
                n193 = call-poly "_DServerSetAttributeValue.vi"("value"=w244, "client request"=w245) -> ()  [unwired: 3 in, 1 out]
              }
              frame "devULongScalar" {
                n194 = call-poly "RandomScalar.vi"() -> ("random value"=w246:u32)  [unwired: 1 in]
                n195 = call-poly "_DServerSetAttributeValue.vi"("value"=w246, "client request"=w247) -> ()  [unwired: 3 in, 1 out]
              }
              frame "devULongSpectrum" {
                n196 = call-poly "Random1DArray.vi"() -> ("array"=w248:u32[])  [unwired: 2 in]
                n197 = call-poly "_DServerSetAttributeValue.vi"("value"=w248, "client request"=w249) -> ()  [unwired: 3 in, 1 out]
              }
              frame "devUShortImage" {
                n198 = call-poly "Random2DArray.vi"() -> ("random array"=w250:u16[][])  [unwired: 2 in]
                n199 = call-poly "_DServerSetAttributeValue.vi"("value"=w250, "client request"=w251) -> ()  [unwired: 3 in, 1 out]
              }
              frame "devUShortScalar" {
                n200 = call-poly "RandomScalar.vi"() -> ("random value"=w252:u16)  [unwired: 1 in]
                n201 = call-poly "_DServerSetAttributeValue.vi"("value"=w252, "client request"=w253) -> ()  [unwired: 3 in, 1 out]
              }
              frame "devUShortSpectrum" {
                n202 = call-poly "Random1DArray.vi"() -> ("array"=w254:u16[])  [unwired: 2 in]
                n203 = call-poly "_DServerSetAttributeValue.vi"("value"=w254, "client request"=w255) -> ()  [unwired: 3 in, 1 out]
              }
              frame "slowReplyAttribute" {
                n204 = stacked-sequence {
                  tunnel: w256 -> [_ w259]
                  frame #0 {
                    # "simulate a slow reply \ngenerating a client \nrequest timeout"
                    n205 = Wait (ms)(milliseconds to wait=u32 3500) -> ()  [unwired: 1 out]
                  }
                  frame #1 {
                    # "simulate a slow reply \ngenerating a client \nrequest timeout"
                    n206 = call-poly "Random1DArray.vi"() -> ("array"=w258:u8[])  [unwired: 2 in]
                    n207 = call-poly "_DServerSetAttributeValue.vi"("value"=w258, "client request"=w259) -> ()  [unwired: 3 in, 1 out]
                  }
                }
              }
              frame "noReplyAttribute" {
                # "we voluntarily don't reply to this request in order to\nobserve the behavior of the tango binding to such a \nsituation - we expect the waiter (i.e. the thread handling \nthe client request to timeout and leave the place) - the \ntango device will block (i.e. will not be able to handle \nanother request) until the timeout expires - we consequently understand easily why we should reply to any single request - the _DServerUnimplementedRequest.vi can be temporary used to deal with \"not yet implemented\" features - see the \"unhandledAttribute\" case for an example"
              }
              frame "unHandledAttribute", Default {
                n208 = call "_DServerUnimplementedRequest.vi"("client request"=w260) -> ()  [unwired: 2 in, 1 out]
              }
            }
          }
          frame "WRITE_ATTR" {
            n209 = call "_DServerUnimplementedRequest.vi"("client request"=w261) -> ()  [unwired: 2 in, 1 out]
          }
          frame "UNKNOWN_REQUEST", Default {
            n210 = call "_DServerUnimplementedRequest.vi"("client request"=w262) -> ()  [unwired: 2 in, 1 out]
          }
        }
        "labview/device/1.1" <- w148
      }
      frame True {
      }
    }
  }
  n211 = while {
    tunnel: w2 -> [w266]
    tunnel: [w265] -> w3
    shift-right: [w275] -> w17
    shift-left: w18 -> [w276]
    shift-right: [w273] -> w15
    shift-left: w14 -> [w274]
    shift-right: [w270] -> w8
    shift-left: w1 -> [w271]
    tunnel: w5 -> [w263]
    tunnel: [w263] -> w4
    stop <- w272 stop-if-true
    n212 = call "_DServerEventHandler.vi"("error in"=w266, "dserver evt."=w263) -> ("error out"=w267:errorcluster, "client request"=w268:T2, "timeout"=w269:bool)  [unwired: 1 in]
    n213 = Or(x="?", y=w267) -> (x .or. y?=w272:bool)
    n214 = case shown="True" w269 {
      tunnel: w268 -> [w280 _]
      tunnel: w276 -> [w286 w315]
      tunnel: [w281 w315] -> w275
      tunnel: w274 -> [w284 w314]
      tunnel: [w285 w314] -> w273
      tunnel: w271 -> [w283 w313]
      tunnel: [w282 w313] -> w270
      tunnel: w267 -> [w278 w312]
      tunnel: [w277 w312] -> w265
      frame False {
        n215 = Unbundle By Name(w280) -> ("Device Name"=w279:string)
        n216 = case shown="\"labview/device/1.1\"" w279 {
          tunnel: w286 -> [w290 w297 w304 w310]
          tunnel: w284 -> [w289 w296 w302 w311]
          tunnel: [w289 w296 w301 w311] -> w285
          tunnel: [w288 w295 w303 w308] -> w282
          tunnel: w283 -> [w288 w295 w303 w309]
          tunnel: [w290 w294 w304 w310] -> w281
          tunnel: w280 -> [_ w293 w300 w307]
          tunnel: w278 -> [w287 w292 w299 w306]
          tunnel: [w287 w291 w298 w305] -> w277
          frame Default {
          }
          frame "labview/device/1.1" {
            n217 = Enqueue Element(queue=w297, element=w293, error in (no error)=w292) -> (queue out=w294:refnum<queue>, error out=w291:errorcluster)  [unwired: 1 in, 1 out]
          }
          frame "labview/device/1.2" {
            n218 = Enqueue Element(queue=w302, element=w300, error in (no error)=w299) -> (queue out=w301:refnum<queue>, error out=w298:errorcluster)  [unwired: 1 in, 1 out]
          }
          frame "labview/device/2.1" {
            n219 = Enqueue Element(queue=w309, element=w307, error in (no error)=w306) -> (queue out=w308:refnum<queue>, error out=w305:errorcluster)  [unwired: 1 in, 1 out]
          }
        }
      }
      frame True {
      }
    }
  }
  n220 = while {
    shift-right: [w316] -> _
    shift-left: w2 -> [w317]
    shift-right: [w318] -> _
    shift-left: w1 -> [w321]
    stop <- w316 stop-if-true
    n221 = Dequeue Element(queue=w321, error in (no error)=w317) -> (queue out=w318:refnum<queue>, element=w320:T2, timed out?=w319:bool, error out=w316:errorcluster)  [unwired: 1 in]
    n222 = case shown="False" w319 {
      tunnel: w320 -> [w322 _]
      frame False {
        n223 = Unbundle By Name(w322) -> ("Request Type"=w323:T3, "Cmd or Attr Name"=w324:string)  [unwired: 1 out]
        n224 = case shown="\"READ_ATTR\"" w323 {
          tunnel: w324 -> [_ w327 _ _]
          tunnel: w322 -> [w325 w326 w434 w435]
          frame "EXEC_CMD" {
            n225 = call "_DServerUnimplementedRequest.vi"("client request"=w325) -> ()  [unwired: 2 in, 1 out]
          }
          frame "READ_ATTR" {
            n226 = case shown="\"devUCharScalar\"" w327 {
              tunnel: w326 -> [w329 w337 w340 w341 w344 w346 w348 w350 w352 w354 w356 w358 w360 w362 w364 w366 w368 w370 w372 w374 w377 w380 w390 w397 w400 w405 w407 w409 w411 w413 w415 w417 w419 w421 w423 w425 w427 w428 w429 _ w433]
              frame "State" {
                n227 = Tick Count (ms)() -> (millisecond timer value=w330:u32)
                n228 = Quotient & Remainder(x=w330, y=u32 2) -> (x-y*floor(x/y)=w332:u32)  [unwired: 1 out]
                n229 = Equal To 0?(x=w332) -> (x = 0?=w331:bool)
                n230 = case shown="True" w331 {
                  tunnel: [_TangoState_t."MOVING" ("Tango Device State") _TangoState_t."STANDBY" ("Tango Device State")] -> w328
                  frame False {
                  }
                  frame True {
                  }
                }
                "Tango Device State 2.1" <- w328
                n231 = call-poly "_DServerSetAttributeValue.vi"("value"=w328, "client request"=w329) -> ()  [unwired: 3 in, 1 out]
              }
              frame "Status" {
                n232 = property on="Tango Device State 2.1" class="Enum (strict)"() -> ("Value"=w336:T1)  [unwired: 2 in, 2 out]
                n233 = call "_TangoStateName.vi"("State"=w336) -> ("State Name"=w338:string)
                n234 = call-poly "_DServerSetAttributeValue.vi"("value"=w338, "client request"=w337) -> ()  [unwired: 3 in, 1 out]
              }
              frame "devBooleanImage" {
                n235 = call-poly "Random2DArray.vi"() -> ("random array"=w339:bool[][])  [unwired: 2 in]
                n236 = call-poly "_DServerSetAttributeValue.vi"("value"=w339, "client request"=w340) -> ()  [unwired: 3 in, 1 out]
              }
              frame "devBooleanScalar" {
                n237 = call-poly "RandomScalar.vi"() -> ("random value"=w342:bool)  [unwired: 1 in]
                n238 = call-poly "_DServerSetAttributeValue.vi"(4:w342, "client request"=w341) -> ()  [unwired: 3 in, 1 out]
              }
              frame "devBooleanSpectrum" {
                n239 = call-poly "Random1DArray.vi"() -> ("array"=w343:bool[])  [unwired: 2 in]
                n240 = call-poly "_DServerSetAttributeValue.vi"("value"=w343, "client request"=w344) -> ()  [unwired: 3 in, 1 out]
              }
              frame "devDoubleImage" {
                n241 = call-poly "Random2DArray.vi"() -> ("random array"=w345:dbl[][])  [unwired: 2 in]
                n242 = call-poly "_DServerSetAttributeValue.vi"("value"=w345, "client request"=w346) -> ()  [unwired: 3 in, 1 out]
              }
              frame "devDoubleScalar" {
                n243 = property on="devDoubleScalar" class="Knob (strict)"() -> ("Value"=w347:dbl)  [unwired: 2 in, 2 out]
                n244 = call-poly "_DServerSetAttributeValue.vi"("value"=w347, "client request"=w348) -> ()  [unwired: 3 in, 1 out]
              }
              frame "devDoubleSpectrum" {
                n245 = call-poly "Random1DArray.vi"() -> ("array"=w349:dbl[])  [unwired: 2 in]
                n246 = call-poly "_DServerSetAttributeValue.vi"("value"=w349, "client request"=w350) -> ()  [unwired: 3 in, 1 out]
              }
              frame "devFloatImage" {
                n247 = call-poly "Random2DArray.vi"() -> ("random array"=w351:sgl[][])  [unwired: 2 in]
                n248 = call-poly "_DServerSetAttributeValue.vi"("value"=w351, "client request"=w352) -> ()  [unwired: 3 in, 1 out]
              }
              frame "devFloatScalar" {
                n249 = call-poly "_DServerSetAttributeValue.vi"("value"=_TangoState_t."RUNNING" ("Tango Device State"), "client request"=w354) -> ()  [unwired: 3 in, 1 out]
              }
              frame "devFloatSpectrum" {
                n250 = call-poly "Random1DArray.vi"() -> ("array"=w355:sgl[])  [unwired: 2 in]
                n251 = call-poly "_DServerSetAttributeValue.vi"("value"=w355, "client request"=w356) -> ()  [unwired: 3 in, 1 out]
              }
              frame "devLong64Image" {
                n252 = call-poly "Random2DArray.vi"() -> ("random array"=w357:i64[][])  [unwired: 2 in]
                n253 = call-poly "_DServerSetAttributeValue.vi"("value"=w357, "client request"=w358) -> ()  [unwired: 3 in, 1 out]
              }
              frame "devLong64Scalar" {
                n254 = call-poly "RandomScalar.vi"() -> ("random value"=w359:i64)  [unwired: 1 in]
                n255 = call-poly "_DServerSetAttributeValue.vi"("value"=w359, "client request"=w360) -> ()  [unwired: 3 in, 1 out]
              }
              frame "devLong64Spectrum" {
                n256 = call-poly "Random1DArray.vi"() -> ("array"=w361:i64[])  [unwired: 2 in]
                n257 = call-poly "_DServerSetAttributeValue.vi"("value"=w361, "client request"=w362) -> ()  [unwired: 3 in, 1 out]
              }
              frame "devLongImage" {
                n258 = call-poly "Random2DArray.vi"() -> ("random array"=w363:i32[][])  [unwired: 2 in]
                n259 = call-poly "_DServerSetAttributeValue.vi"("value"=w363, "client request"=w364) -> ()  [unwired: 3 in, 1 out]
              }
              frame "devLongScalar" {
                n260 = call-poly "RandomScalar.vi"() -> ("random value"=w365:i32)  [unwired: 1 in]
                n261 = call-poly "_DServerSetAttributeValue.vi"("value"=w365, "client request"=w366) -> ()  [unwired: 3 in, 1 out]
              }
              frame "devLongSpectrum" {
                n262 = call-poly "Random1DArray.vi"() -> ("array"=w367:i32[])  [unwired: 2 in]
                n263 = call-poly "_DServerSetAttributeValue.vi"("value"=w367, "client request"=w368) -> ()  [unwired: 3 in, 1 out]
              }
              frame "devShortImage" {
                n264 = call-poly "Random2DArray.vi"() -> ("random array"=w369:i16[][])  [unwired: 2 in]
                n265 = call-poly "_DServerSetAttributeValue.vi"("value"=w369, "client request"=w370) -> ()  [unwired: 3 in, 1 out]
              }
              frame "devShortScalar" {
                n266 = call-poly "RandomScalar.vi"() -> ("random value"=w371:i16)  [unwired: 1 in]
                n267 = call-poly "_DServerSetAttributeValue.vi"("value"=w371, "client request"=w372) -> ()  [unwired: 3 in, 1 out]
              }
              frame "devShortSpectrum" {
                n268 = call-poly "Random1DArray.vi"() -> ("array"=w373:i16[])  [unwired: 2 in]
                n269 = call-poly "_DServerSetAttributeValue.vi"("value"=w373, "client request"=w374) -> ()  [unwired: 3 in, 1 out]
              }
              frame "devStateImage" {
                n270 = property on="Tango Device State 2.1" class="Enum (strict)"() -> ("Value"=w376:T1)  [unwired: 2 in, 2 out]
                n271 = Initialize Array(w376, 32 ("dimension size"), 32 ("dimension size")) -> (w375:T1[][])
                n272 = call-poly "_DServerSetAttributeValue.vi"("value"=w375, "client request"=w377) -> ()  [unwired: 3 in, 1 out]
              }
              frame "devStateScalar" {
                n273 = Tick Count (ms)() -> (millisecond timer value=w382:u32)
                n274 = Quotient & Remainder(x=w382, y=u32 2) -> (x-y*floor(x/y)=w384:u32)  [unwired: 1 out]
                n275 = Equal To 0?(x=w384) -> (x = 0?=w383:bool)
                n276 = case shown="False" w383 {
                  tunnel: [_TangoState_t."STANDBY" ("Tango Device State") _TangoState_t."RUNNING" ("Tango Device State")] -> w381
                  frame False {
                  }
                  frame True {
                  }
                }
                n277 = call-poly "_DServerSetAttributeValue.vi"("value"=w381, "client request"=w380) -> ()  [unwired: 3 in, 1 out]
              }
              frame "devStateSpectrum" {
                n278 = property on="Tango Device State 2.1" class="Enum (strict)"() -> ("Value"=w389:T1)  [unwired: 2 in, 2 out]
                n279 = Initialize Array(w389, 32 ("dimension size")) -> (w388:T1[])
                n280 = call-poly "_DServerSetAttributeValue.vi"("value"=w388, "client request"=w390) -> ()  [unwired: 3 in, 1 out]
              }
              frame "devStringImage" {
                n281 = call "RandomValue.vi"() -> ("random value"=w395:dbl)  [unwired: 1 in]
                n282 = Number To Hexadecimal String(2:w395) -> (0:w394:string)  [unwired: 1 in]
                n283 = Initialize Array(w394, 32 ("dimension size"), 32 ("dimension size")) -> (w393:string[][])
                n284 = call-poly "_DServerSetAttributeValue.vi"("value"=w393, "client request"=w397) -> ()  [unwired: 3 in, 1 out]
              }
              frame "devStringScalar" {
                n285 = call "RandomValue.vi"() -> ("random value"=w399:dbl)  [unwired: 1 in]
                n286 = Number To Hexadecimal String(2:w399) -> (0:w398:string)  [unwired: 1 in]
                n287 = call-poly "_DServerSetAttributeValue.vi"("value"=w398, "client request"=w400) -> ()  [unwired: 3 in, 1 out]
              }
              frame "devStringSpectrum" {
                n288 = call "RandomValue.vi"() -> ("random value"=w403:dbl)  [unwired: 1 in]
                n289 = Number To Hexadecimal String(2:w403) -> (0:w402:string)  [unwired: 1 in]
                n290 = Initialize Array(w402, 32 ("dimension size")) -> (w401:string[])
                n291 = call-poly "_DServerSetAttributeValue.vi"("value"=w401, "client request"=w405) -> ()  [unwired: 3 in, 1 out]
              }
              frame "devUCharImage" {
                n292 = call-poly "Random2DArray.vi"() -> ("random array"=w406:u8[][])  [unwired: 2 in]
                n293 = call-poly "_DServerSetAttributeValue.vi"("value"=w406, "client request"=w407) -> ()  [unwired: 3 in, 1 out]
              }
              frame "devUCharScalar" {
                n294 = call-poly "RandomScalar.vi"() -> ("random value"=w408:u8)  [unwired: 1 in]
                n295 = call-poly "_DServerSetAttributeValue.vi"("value"=w408, "client request"=w409) -> ()  [unwired: 3 in, 1 out]
              }
              frame "devUCharSpectrum" {
                n296 = call-poly "Random1DArray.vi"() -> ("array"=w410:u8[])  [unwired: 2 in]
                n297 = call-poly "_DServerSetAttributeValue.vi"("value"=w410, "client request"=w411) -> ()  [unwired: 3 in, 1 out]
              }
              frame "devULong64Image" {
                n298 = call-poly "Random2DArray.vi"() -> ("random array"=w412:i64[][])  [unwired: 2 in]
                n299 = call-poly "_DServerSetAttributeValue.vi"("value"=w412, "client request"=w413) -> ()  [unwired: 3 in, 1 out]
              }
              frame "devULong64Scalar" {
                n300 = call-poly "RandomScalar.vi"() -> ("random value"=w414:u64)  [unwired: 1 in]
                n301 = call-poly "_DServerSetAttributeValue.vi"("value"=w414, "client request"=w415) -> ()  [unwired: 3 in, 1 out]
              }
              frame "devULong64Spectrum" {
                n302 = call-poly "Random1DArray.vi"() -> ("array"=w416:u64[])  [unwired: 2 in]
                n303 = call-poly "_DServerSetAttributeValue.vi"("value"=w416, "client request"=w417) -> ()  [unwired: 3 in, 1 out]
              }
              frame "devULongImage" {
                n304 = call-poly "Random2DArray.vi"() -> ("random array"=w418:u32[][])  [unwired: 2 in]
                n305 = call-poly "_DServerSetAttributeValue.vi"("value"=w418, "client request"=w419) -> ()  [unwired: 3 in, 1 out]
              }
              frame "devULongScalar" {
                n306 = call-poly "RandomScalar.vi"() -> ("random value"=w420:u32)  [unwired: 1 in]
                n307 = call-poly "_DServerSetAttributeValue.vi"("value"=w420, "client request"=w421) -> ()  [unwired: 3 in, 1 out]
              }
              frame "devULongSpectrum" {
                n308 = call-poly "Random1DArray.vi"() -> ("array"=w422:u32[])  [unwired: 2 in]
                n309 = call-poly "_DServerSetAttributeValue.vi"("value"=w422, "client request"=w423) -> ()  [unwired: 3 in, 1 out]
              }
              frame "devUShortImage" {
                n310 = call-poly "Random2DArray.vi"() -> ("random array"=w424:u16[][])  [unwired: 2 in]
                n311 = call-poly "_DServerSetAttributeValue.vi"("value"=w424, "client request"=w425) -> ()  [unwired: 3 in, 1 out]
              }
              frame "devUShortScalar" {
                n312 = call-poly "RandomScalar.vi"() -> ("random value"=w426:u16)  [unwired: 1 in]
                n313 = call-poly "_DServerSetAttributeValue.vi"("value"=w426, "client request"=w427) -> ()  [unwired: 3 in, 1 out]
              }
              frame "devUShortSpectrum" {
                n314 = call-poly "Random1DArray.vi"() -> ()  [unwired: 2 in, 1 out]
                n315 = call-poly "_DServerSetAttributeValue.vi"("client request"=w428) -> ()  [unwired: 4 in, 1 out]
              }
              frame "slowReplyAttribute" {
                n316 = stacked-sequence {
                  tunnel: w429 -> [_ w432]
                  frame #0 {
                    # "simulate a slow reply \ngenerating a client \nrequest timeout"
                    n317 = Wait (ms)(milliseconds to wait=u32 3500) -> ()  [unwired: 1 out]
                  }
                  frame #1 {
                    # "simulate a slow reply \ngenerating a client \nrequest timeout"
                    n318 = call-poly "Random1DArray.vi"() -> ("array"=w431:u8[])  [unwired: 2 in]
                    n319 = call-poly "_DServerSetAttributeValue.vi"("value"=w431, "client request"=w432) -> ()  [unwired: 3 in, 1 out]
                  }
                }
              }
              frame "noReplyAttribute" {
                # "we voluntarily don't reply to this request in order to\nobserve the behavior of the tango binding to such a \nsituation - we expect the waiter (i.e. the thread handling \nthe client request to timeout and leave the place) - the \ntango device will block (i.e. will not be able to handle \nanother request) until the timeout expires - we consequently understand easily why we should reply to any single request - the _DServerUnimplementedRequest.vi can be temporary used to deal with \"not yet implemented\" features - see the \"unhandledAttribute\" case for an example"
              }
              frame "unHandledAttribute", Default {
                n320 = call "_DServerUnimplementedRequest.vi"("client request"=w433) -> ()  [unwired: 2 in, 1 out]
              }
            }
          }
          frame "WRITE_ATTR" {
            n321 = call "_DServerUnimplementedRequest.vi"("client request"=w434) -> ()  [unwired: 2 in, 1 out]
          }
          frame "UNKNOWN_REQUEST", Default {
            n322 = call "_DServerUnimplementedRequest.vi"("client request"=w435) -> ()  [unwired: 2 in, 1 out]
          }
        }
        "labview/device/2.1" <- w322
      }
      frame True {
      }
    }
  }
  n323 = call "_DServerStop.vi"("error in"=w3, "dserver evt."=w4) -> ()  [unwired: 1 in, 1 out]
  n324 = Release Queue(queue=w17, error in (no error)=w3) -> ()  [unwired: 1 in, 3 out]
  n325 = Release Queue(queue=w15, error in (no error)=w3) -> ()  [unwired: 1 in, 3 out]
  n326 = Release Queue(queue=w8, error in (no error)=w3) -> ()  [unwired: 1 in, 3 out]
